vi "TestJDebug.vi"() -> ()   [LabVIEW 2009]
panel:
  out "output cluster":T1
  in  "file path (use dialog)":path
  in  "FPGA IP Address":string
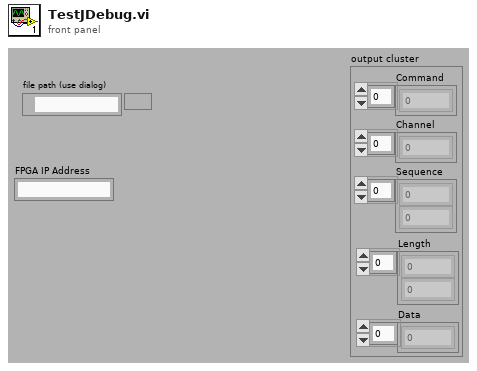
[diagram p1: front panel]
types:
  T1 = cluster{"Command":i32[], "Channel":i32[], "Sequence":i32[], "Length":i32[], "Data":i32[]}
  T2 = enum16{"open", "replace", "create", "open or create", "replace or create", "replace or create with confirmation"}
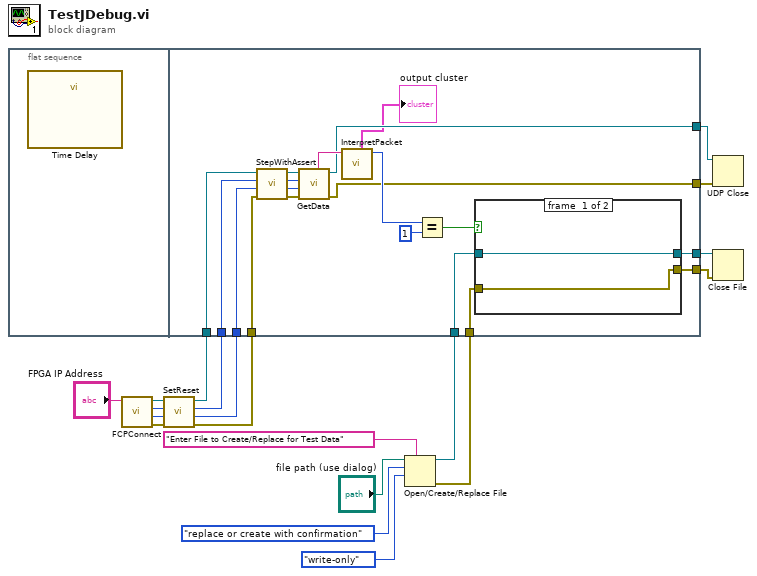
[diagram p0: block diagram]
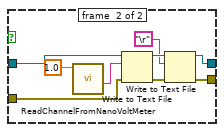
[diagram p2: hidden frame]
diagram:
  n1 = flat-sequence {
    tunnel: w14 -> [w38]
    tunnel: w13 -> [w37]
    tunnel: w12 -> [w36]
    tunnel: w11 -> [w35]
    tunnel: [w21] -> w10
    tunnel: [w22] -> w9
    tunnel: w4 -> [w26]
    tunnel: w3 -> [w25]
    tunnel: [w24] -> w2
    tunnel: [w23] -> w1
    frame #0 {
      n2 = call "Time Delay"() -> ()  [unwired: 11 in, 1 out]
    }
    frame #1 {
      n3 = call "StepWithAssert.vi"("error in (no error)"=w35, "SequenceNumber"=w36, "address"=w37, "connection ID"=w38) -> ("error out"=w30:errorcluster, "SequenceNumber out"=w31:i32, "address out"=w32:u32, "connection ID out"=w33:refnum<k16>)  [unwired: 4 in]
      n4 = call "GetData.vi"("error in (no error)"=w30, "SequenceNumber"=w31, "address"=w32, "connection ID"=w33) -> ("error out"=w22:errorcluster, "connection ID out"=w21:refnum<k16>, "data out"=w29:string)  [unwired: 3 in, 2 out]
      n5 = call "InterpretPacket.vi"("Data In"=w29) -> ("Data Out"=w28:u8, "output cluster"=→"output cluster":T1)  [unwired: 9 in]
      n6 = Equal?(x=w28, y=u8 1) -> (x = y?=w27:bool)
      n7 = case shown="False" w27 {
        tunnel: w26 -> [w40 w47]
        tunnel: w25 -> [w39 w46]
        tunnel: [w40 w42] -> w24
        tunnel: [w39 w41] -> w23
        frame #0 {
        }
        frame #1 {
          n8 = call "ReadChannelFromNanoVoltMeter.vi"("ChannelSelection"=1.0) -> ("String Measurement"=w48:string)  [unwired: 8 in, 2 out]
          n9 = Write to Text File(file (use dialog)=w47, text=w48, error in=w46) -> (refnum out=w45:refnum<file>, error out=w44:errorcluster)  [unwired: 1 in, 1 out]
          n10 = Write to Text File(file (use dialog)=w45, text="\r", error in=w44) -> (refnum out=w42:refnum<file>, error out=w41:errorcluster)  [unwired: 1 in, 1 out]
        }
      }
    }
  }
  n11 = call "FCPConnect.vi"("FPGA IP Address"="FPGA IP Address") -> ("error out"=w17:errorcluster, "Sequence Number"=w15:i32, "FPGA IP Address Out"=w16:u32, "connection ID out"=w18:refnum<k16>)  [unwired: 7 in]
  n12 = call "SetReset.vi"("error in (no error)"=w17, "SequenceNumber"=w15, "address"=w16, "connection ID"=w18) -> ("error out"=w11:errorcluster, "SequenceNumber out"=w12:i32, "Address out"=w13:u32, "connection ID out"=w14:refnum<k16>)  [unwired: 4 in]
  n13 = Open/Create/Replace File(file path (use dialog)="file path (use dialog)", prompt="Enter File to Create/Replace for Test Data", operation (0:open)=T2."replace or create with confirmation", access (0:read/write)=enum16{"read/write", "read-only", "write-only"}."write-only") -> (refnum out=w4:refnum<file>, error out=w3:errorcluster)  [unwired: 2 in, 1 out]
  n14 = UDP Close(connection ID=w10, 8:w9) -> ()  [unwired: 2 out]
  n15 = Close File(refnum=w2, error in=w1) -> ()  [unwired: 2 out]
